vi "New.vi"(8 "error in (no error)":errorcluster, 11 "MsgPack Data":string) -> (0 "error out":errorcluster, 3 "Deserializer":refnum<class "MsgPackDeserializer.lvclass">)   [LabVIEW 2015, in "MsgPackDeserializer.lvclass"]
uses:
  MsgPackDeserializer.lvclass
  MsgPackDeserializer.lvclass/MsgPackDeserializer.ctl
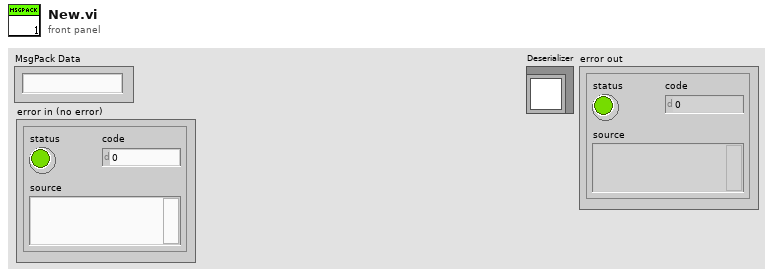
[diagram p1: front panel]
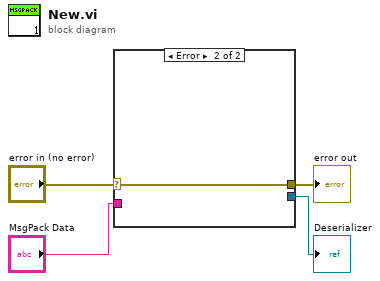
[diagram p0: block diagram]
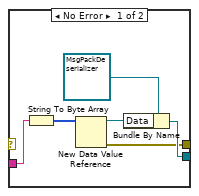
[diagram p2: hidden frame]
diagram:
  n1 = case shown="Error" "error in (no error)" {
    selector: "error in (no error)" -> [_ w11]
    tunnel: "MsgPack Data" -> [w10 _]
    tunnel: [w6 _] -> w3
    tunnel: [w5 w11] -> w2
    frame No Error {
      n2 = String To Byte Array(string=w10) -> (unsigned byte array=w9:u8[])
      n3 = New Data Value Reference(data value=w9) -> (data value reference=w7:refnum<data-value>, error out=w5:errorcluster)  [unwired: 1 in]
      n4 = Bundle By Name(cluster=refnum<class "MsgPackDeserializer.lvclass"> refnum ("MsgPackDeserializer.lvclass"), "Data"=w7) -> (w6:refnum<class "MsgPackDeserializer.lvclass">)
    }
    frame Error {
    }
  }
  "Deserializer" <- w3
  "error out" <- w2
